vi "Test.vi"() -> ()   [LabVIEW 2018, in "Bronkhorst M13 Flow Meter.lvlib"]
uses:
  Bronkhorst M13 Flow Meter.lvlib
  Settings Cluster.ctl
panel:
  in  "stop":bool
  in  "error in (no error)":errorcluster
  out "Temp (C)":sgl
  out "flow":dbl
  out "Density kg/m^3":sgl
  in  "Bronkhorst Settings in":T1={"VISA resource name"="", "Simulated?"=FALSE, "Smoothing Steps"=1} {"Smoothing Steps" min=1 step=1}
  out "error out":errorcluster
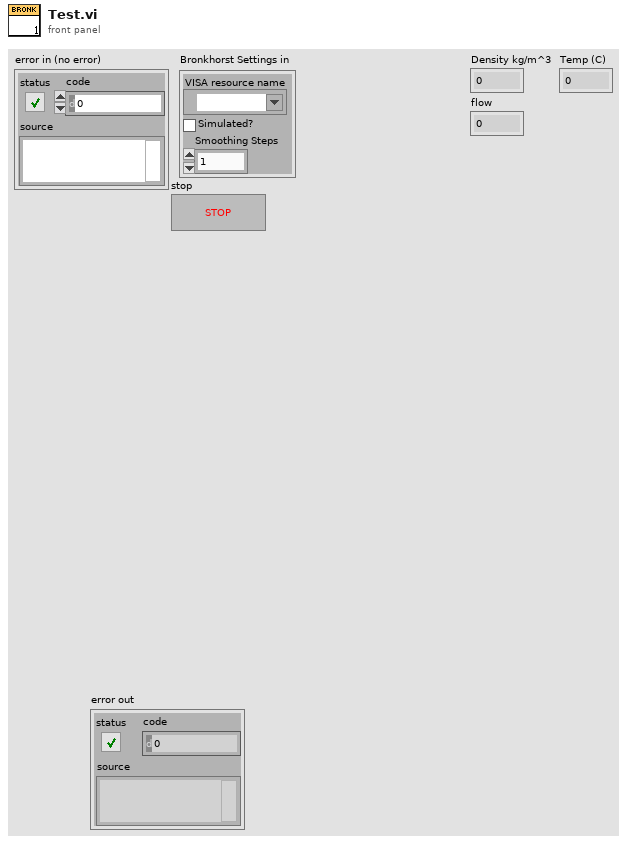
[diagram p1: front panel]
types:
  T1 = typedef "Bronkhorst M13 Flow Meter.lvlib/Settings Cluster.ctl" = cluster{"VISA resource name":refnum<visa-resource-name>, "Simulated?":bool, "Smoothing Steps":i32}
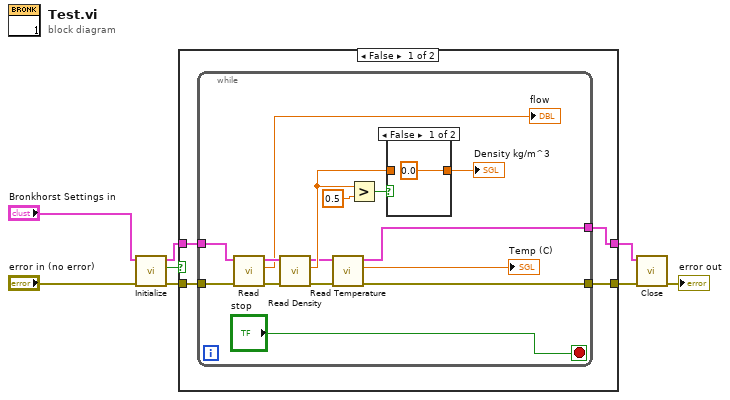
[diagram p0: block diagram]
diagram:
  n1 = call "Initialize.vi"("error in (no error)"="error in (no error)", "Bronkhorst Settings in"="Bronkhorst Settings in") -> ("error out"=w4:errorcluster, "No Meter Connnected"=w3:bool, "Bronkhorst Settings out"=w6:T1)  [unwired: 7 in]
  n2 = case shown="False" w3 {
    tunnel: [w12 w31] -> w2
    tunnel: [w11 w30] -> w8
    tunnel: w6 -> [w10 w30]
    tunnel: w4 -> [w9 w31]
    frame False {
      n3 = while {
        tunnel: [w27] -> w12
        tunnel: w10 -> [w26]
        tunnel: w9 -> [w15]
        tunnel: [w14] -> w11
        stop <- "stop" stop-if-true
        n4 = call "Read.vi"("error in (no error)"=w15, "Bronkhorst Settings in"=w26) -> ("error out"=w24:errorcluster, "flow"=→"flow":dbl, "Bronkhorst Settings out"=w25:T1)  [unwired: 6 in, 1 out]
        n5 = call "Read Density.vi"("error in (no error)"=w24, "Bronkhorst Settings in"=w25) -> ("error out"=w20:errorcluster, "Density kg/m^3"=w21:sgl, "Bronkhorst Settings out"=w19:T1)  [unwired: 6 in, 1 out]
        n6 = call "Read Temperature.vi"("error in (no error)"=w20, "Bronkhorst Settings in"=w19) -> ("error out"=w27:errorcluster, "Temp (C)"=→"Temp (C)":sgl, "Bronkhorst Settings out"=w14:T1)  [unwired: 6 in, 1 out]
        n7 = Greater?(x=w21, y=0.5) -> (0:w22:bool)
        n8 = case shown="False" w22 {
          tunnel: [sgl 0.0 ("Density kg/m^3") w29] -> w18
          tunnel: w21 -> [_ w29]
          frame False {
          }
          frame True {
          }
        }
        "Density kg/m^3" <- w18
      }
    }
    frame True {
    }
  }
  n9 = call "Close.vi"("error in (no error)"=w2, "Bronkhorst Settings in"=w8) -> ("error out"=→"error out":errorcluster)  [unwired: 8 in, 1 out]
